vi "ALARM MAIN.vi"(8 "Array soglie interpolate in":T2[](array[typedef]), 9 "Array soglie costanti in":T1[](array[typedef]), 10 "new data":T3, 11 "old data":T3) -> (0 "Array soglie interpolate out":T2[](array[typedef]), 1 "Array soglie costanti out":T1[](array[typedef]), 2 "alarm error":errorcluster, 3 "DATA OUT":cluster{T1[], T2[]}, 4 "AGGIORNA?":bool)   [LabVIEW 2019]
uses:
  TypeDef/cluster allarme interp.ctl
  TypeDef/cluster allarme cost.ctl
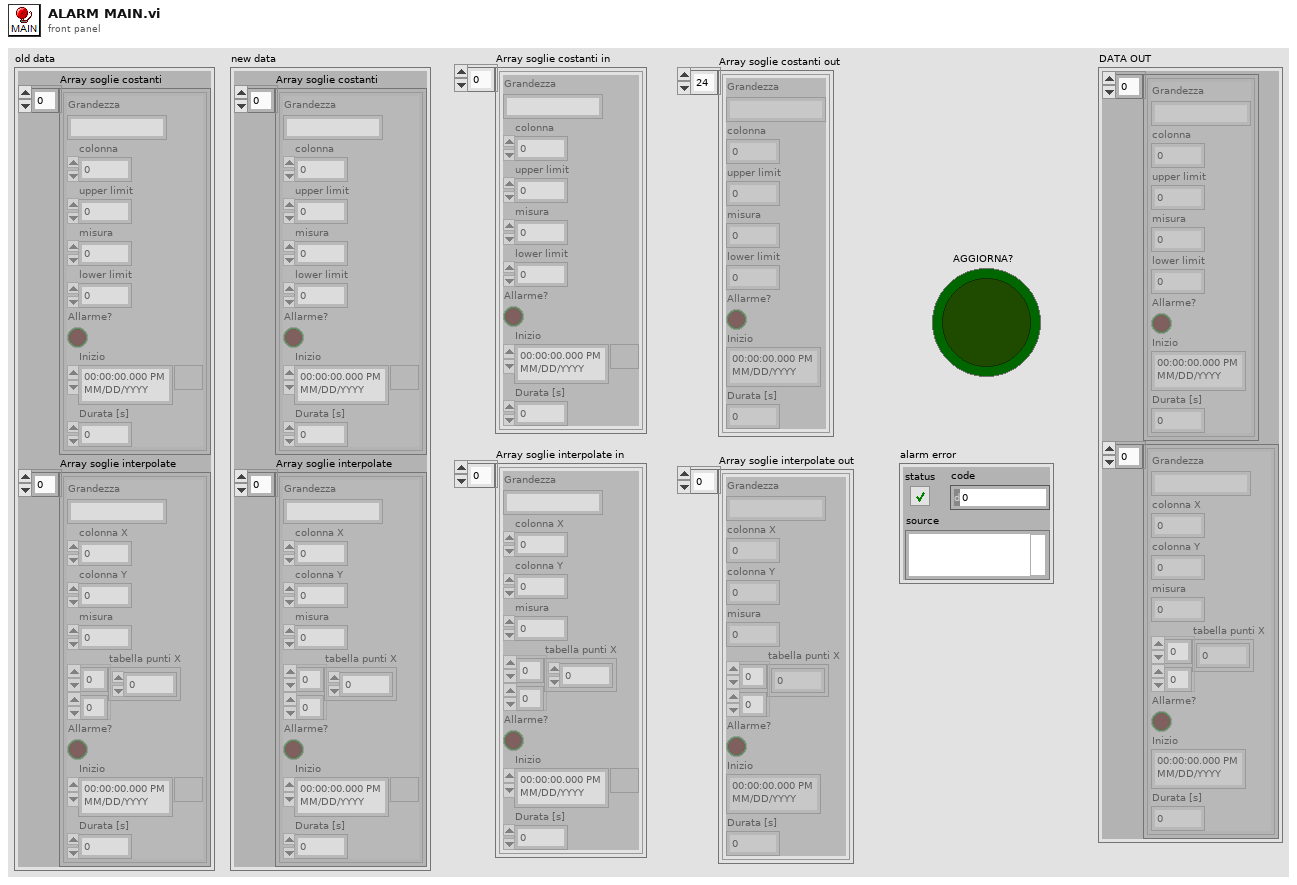
[diagram p1: front panel]
types:
  T1 = typedef "cluster allarme cost.ctl" = cluster{"Grandezza":string, "colonna":i32, "upper limit":dbl, "misura":dbl, "lower limit":dbl, "Allarme?":bool, "Inizio":timestamp, "Durata [s]":dbl}
  T2 = typedef "cluster allarme interp.ctl" = cluster{"Grandezza":string, "colonna X":i32, "colonna Y":i32, "misura":dbl, "tabella punti X":dbl[][], "Allarme?":bool, "Inizio":timestamp, "Durata [s]":dbl}
  T3 = cluster{"Array soglie costanti":T1[], "Array soglie interpolate":T2[]}
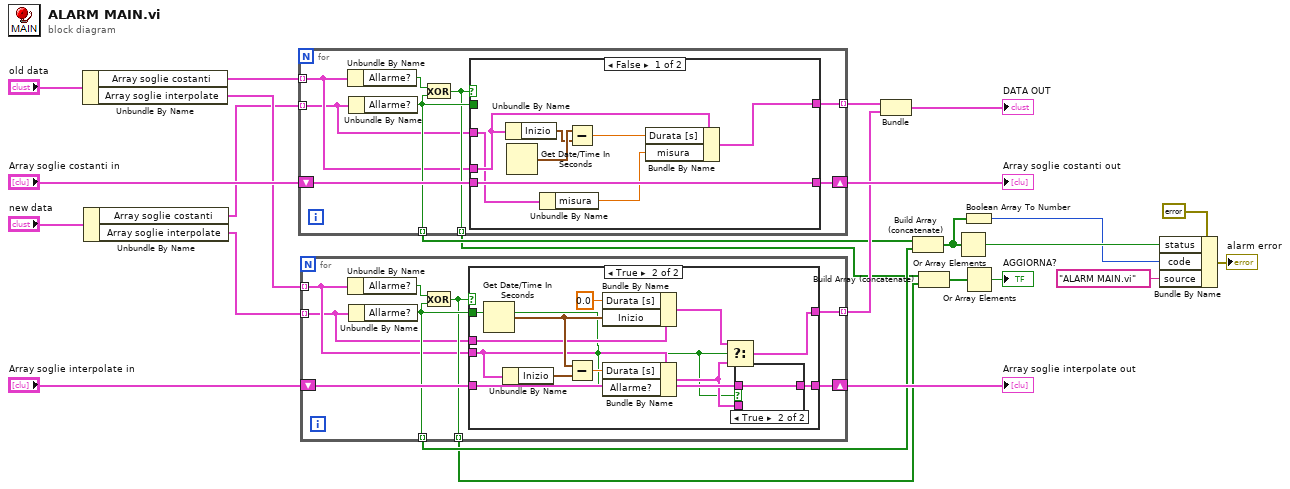
[diagram p0: block diagram]
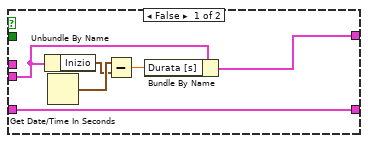
[diagram p2: hidden frame]
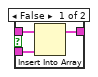
[diagram p3: hidden frame]
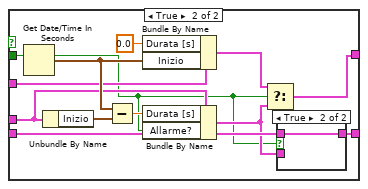
[diagram p4: hidden frame]
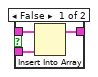
[diagram p5: hidden frame]
diagram:
  n1 = Unbundle By Name("old data") -> ("Array soglie costanti"=w16:T1[], "Array soglie interpolate"=w17:T2[])
  n2 = Unbundle By Name("new data") -> ("Array soglie costanti"=w14:T1[], "Array soglie interpolate"=w18:T2[])
  n3 = for {
    tunnel: w14 -> [w26] mode=indexing
    tunnel: w16 -> [w27] mode=indexing
    tunnel: [w32] -> w19 mode=indexing
    shift-right: [w30] -> w23
    shift-left: "Array soglie costanti in" -> [w31]
    tunnel: [w29] -> w12 mode=indexing
    tunnel: [w28] -> w7 mode=indexing
    n4 = Unbundle By Name(w27) -> ("Allarme?"=w33:bool)
    n5 = Unbundle By Name(w26) -> ("Allarme?"=w29:bool)
    n6 = Exclusive Or(1:w29, 2:w33) -> (0:w28:bool)
    n7 = case shown="False" w28 {
      tunnel: w29 -> [_ w42]
      tunnel: w27 -> [w40 w44]
      tunnel: [w36 w50] -> w32
      tunnel: w31 -> [w39 w49]
      tunnel: [w39 w48] -> w30
      tunnel: w26 -> [w35 w43]
      frame False {
        n8 = Unbundle By Name(w40) -> ("Inizio"=w37:timestamp)
        n9 = Get Date/Time In Seconds() -> (seconds since 1Jan1904=w38:timestamp)
        n10 = Unbundle By Name(w35) -> ("misura"=w34:dbl)
        n11 = Subtract(x=w38, y=w37) -> (x-y=w41:dbl)
        n12 = Bundle By Name(cluster=w40, "Durata [s]"=w41, "misura"=w34) -> (w36:T1)
      }
      frame True {
        n13 = Get Date/Time In Seconds() -> (seconds since 1Jan1904=w47:timestamp)
        n14 = Unbundle By Name(w44) -> ("Inizio"=w46:timestamp)
        n15 = Subtract(x=w47, y=w46) -> (x-y=w52:dbl)
        n16 = Bundle By Name(cluster=w43, "Durata [s]"=0.0, "Inizio"=w47) -> (w51:T1)
        n17 = Bundle By Name(cluster=w44, "Durata [s]"=w52, "Allarme?"=w42) -> (w45:T1)
        n18 = Select(t=w51, s=w42, f=w45) -> (s? t:f=w50:T1)
        n19 = case shown="True" w42 {
          tunnel: w49 -> [w56 w57]
          tunnel: [w55 w57] -> w48
          tunnel: w45 -> [w54 _]
          frame False {
            n20 = Insert Into Array(array=w56, new element=w54) -> (w55:T1[])  [unwired: 1 in]
          }
          frame True {
          }
        }
      }
    }
  }
  "Array soglie costanti out" <- w23
  n21 = for {
    tunnel: w18 -> [w58] mode=indexing
    tunnel: w17 -> [w59] mode=indexing
    tunnel: [w64] -> w20 mode=indexing
    shift-right: [w62] -> w25
    shift-left: "Array soglie interpolate in" -> [w63]
    tunnel: [w61] -> w11 mode=indexing
    tunnel: [w60] -> w8 mode=indexing
    n22 = Unbundle By Name(w59) -> ("Allarme?"=w65:bool)
    n23 = Unbundle By Name(w58) -> ("Allarme?"=w61:bool)
    n24 = Exclusive Or(1:w61, 2:w65) -> (0:w60:bool)
    n25 = case shown="True" w60 {
      tunnel: w61 -> [_ w72]
      tunnel: w59 -> [w70 w74]
      tunnel: [w66 w80] -> w64
      tunnel: w63 -> [w69 w79]
      tunnel: [w69 w78] -> w62
      tunnel: w58 -> [_ w73]
      frame False {
        n26 = Unbundle By Name(w70) -> ("Inizio"=w67:timestamp)
        n27 = Get Date/Time In Seconds() -> (seconds since 1Jan1904=w68:timestamp)
        n28 = Subtract(x=w68, y=w67) -> (x-y=w71:dbl)
        n29 = Bundle By Name(cluster=w70, "Durata [s]"=w71) -> (w66:T2)
      }
      frame True {
        n30 = Get Date/Time In Seconds() -> (seconds since 1Jan1904=w77:timestamp)
        n31 = Unbundle By Name(w74) -> ("Inizio"=w76:timestamp)
        n32 = Subtract(x=w77, y=w76) -> (x-y=w82:dbl)
        n33 = Bundle By Name(cluster=w73, "Durata [s]"=0.0, "Inizio"=w77) -> (w81:T2)
        n34 = Bundle By Name(cluster=w74, "Durata [s]"=w82, "Allarme?"=w72) -> (w75:T2)
        n35 = Select(t=w81, s=w72, f=w75) -> (s? t:f=w80:T2)
        n36 = case shown="True" w72 {
          tunnel: w79 -> [w86 w87]
          tunnel: [w85 w87] -> w78
          tunnel: w75 -> [w84 _]
          frame False {
            n37 = Insert Into Array(array=w86, new element=w84) -> (w85:T2[])  [unwired: 1 in]
          }
          frame True {
          }
        }
      }
    }
  }
  "Array soglie interpolate out" <- w25
  n38 = Bundle(w19, w20) -> (→"DATA OUT":cluster{T1[], T2[]})  [unwired: 1 in]
  n39 = Build Array (concatenate)(w12, w11) -> (w4:bool[])
  n40 = Build Array (concatenate)(w7, w8) -> (w9:bool[])
  n41 = Or Array Elements(Boolean array=w4) -> (logical OR=w5:bool)
  n42 = Boolean Array To Number(Boolean array=w4) -> (number=w3:u32)
  n43 = Or Array Elements(Boolean array=w9) -> (logical OR=→"AGGIORNA?":bool)
  n44 = Bundle By Name(cluster=errorcluster {"status"=FALSE, "code"=0, "source"=""} ("error constant"), "status"=w5, "code"=w3, "source"="ALARM MAIN.vi") -> (→"alarm error":errorcluster)
